vi "Create Serial Output Channel CSI-2 IO x8.vi"() -> (4 "serial output channel io x8":T4)   [LabVIEW 2020, in "GettingStarted_Gen_148X_FPGA.lvlib"]
uses:
  GettingStarted_Gen_148X_FPGA.lvlib
  Common/Types/Serial Output Channel IO.ctl
  Common/Types/Serial Output Channel IO 32b.ctl
  Common/Types/Serial Output Channel IO 64b.ctl
  Common/GettingStarted_Common_148X_FPGA.lvlib
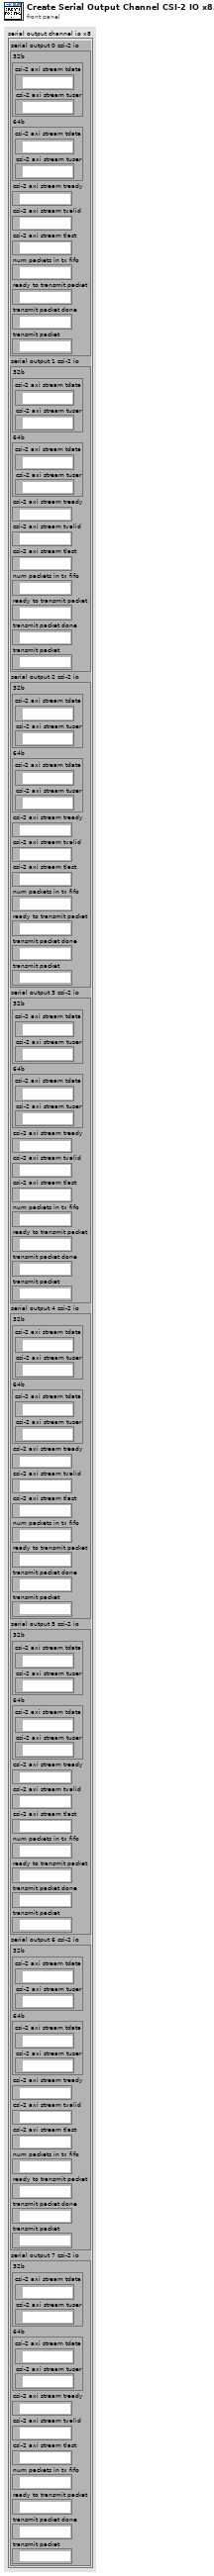
[diagram p1: front panel]
types:
  T1 = typedef "GettingStarted_Common_148X_FPGA.lvlib/Serial Output Channel IO.ctl" = cluster{"32b":T2, "64b":T3, "csi-2 axi stream tready":refnum<k21>, "csi-2 axi stream tvalid":refnum<k21>, "csi-2 axi stream tlast":refnum<k21>, "num packets in tx fifo":refnum<k21>, "ready to transmit packet":refnum<k21>, "transmit packet done":refnum<k21>, "transmit packet":refnum<k21>}
  T2 = typedef "GettingStarted_Common_148X_FPGA.lvlib/Serial Output Channel IO 32b.ctl" = cluster{"csi-2 axi stream tdata":refnum<k21>, "csi-2 axi stream tuser":refnum<k21>}
  T3 = typedef "GettingStarted_Common_148X_FPGA.lvlib/Serial Output Channel IO 64b.ctl" = cluster{"csi-2 axi stream tdata":refnum<k21>, "csi-2 axi stream tuser":refnum<k21>}
  T4 = cluster{"serial output 0 csi-2 io":T1, "serial output 1 csi-2 io":T1, "serial output 2 csi-2 io":T1, "serial output 3 csi-2 io":T1, "serial output 4 csi-2 io":T1, "serial output 5 csi-2 io":T1, "serial output 6 csi-2 io":T1, "serial output 7 csi-2 io":T1}
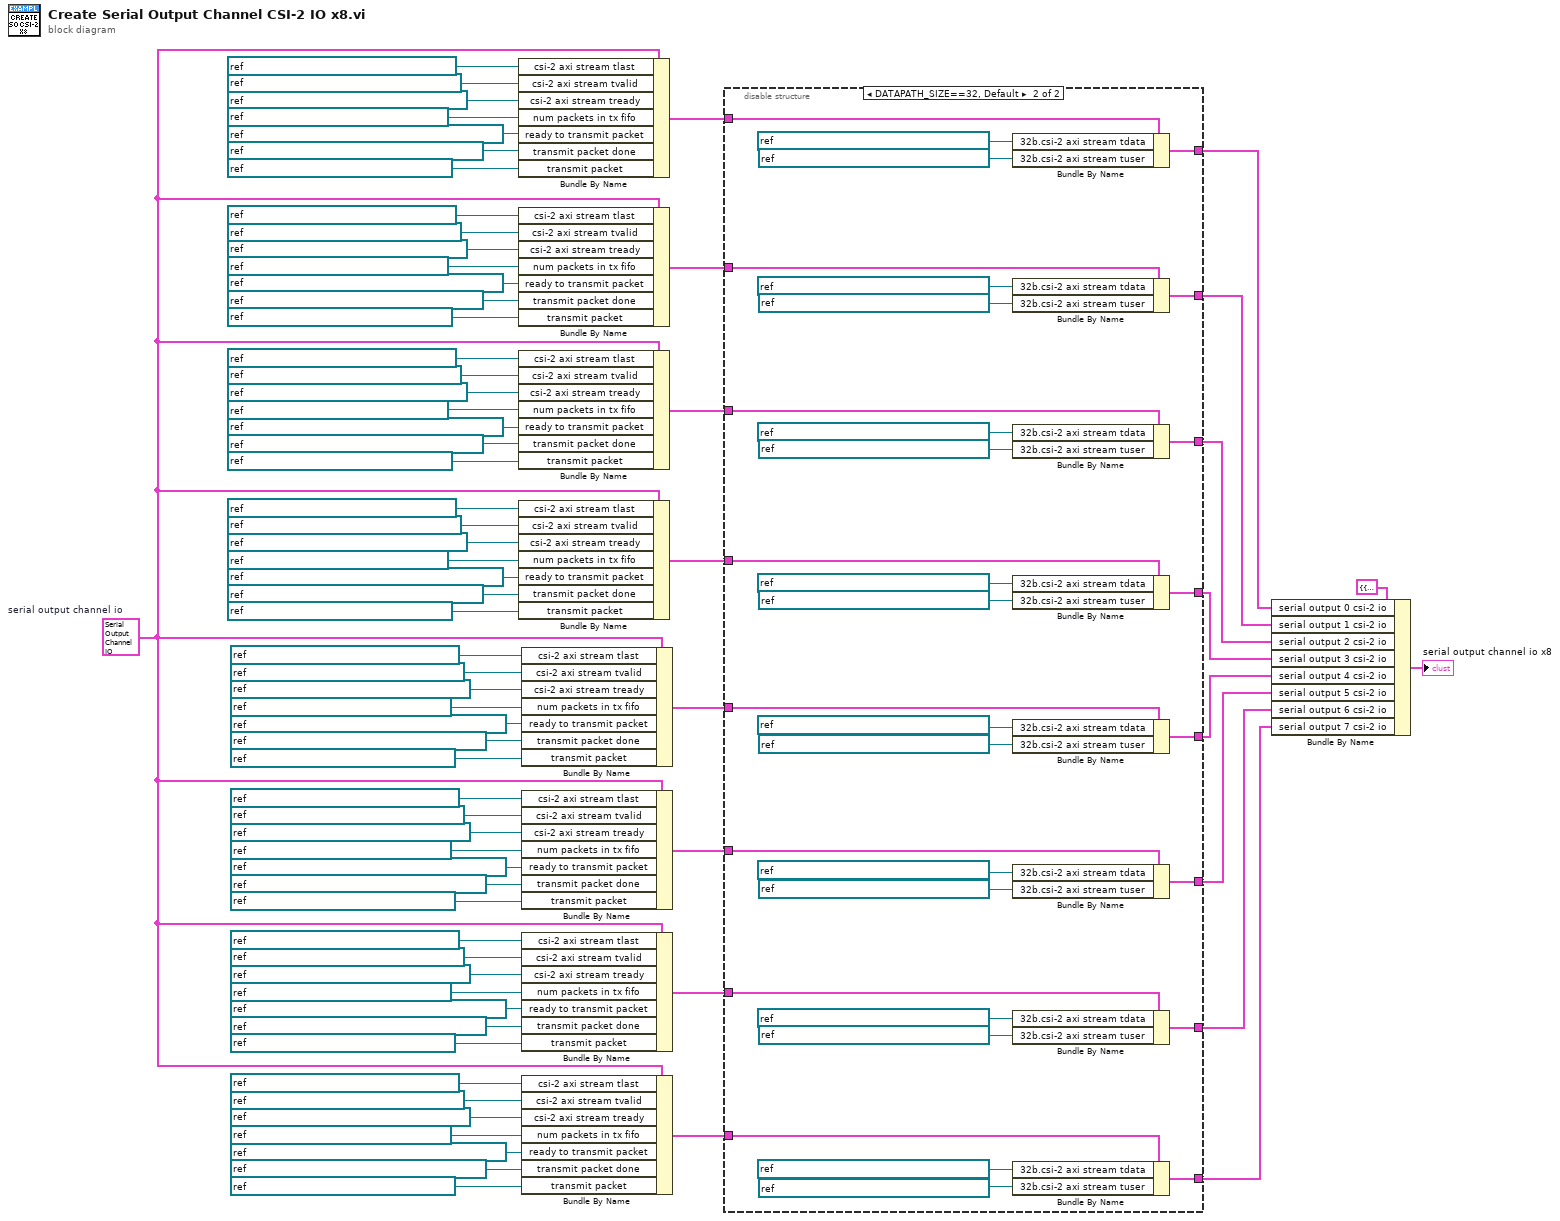
[diagram p0: block diagram]
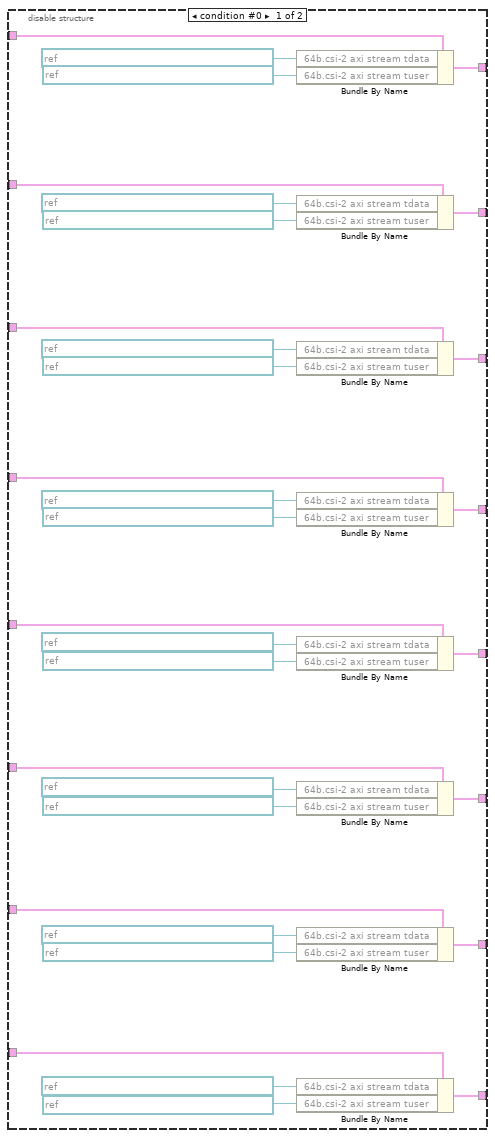
[diagram p2: hidden frame]
diagram:
  w21 = T1 {"32b"={"csi-2 axi stream tdata"="", "csi-2 axi stream tuser"=""}, "64b"={"csi-2 axi stream tdata"="", "csi-2 axi stream tuser"=""}, "csi-2 axi stream tready"="", "csi-2 axi stream tvalid"="", "csi-2 axi stream tlast"="", "num packets in tx fifo"="", "ready to transmit packet"="", "transmit packet done"="", "transmit packet"=""}  # serial output channel io
  n1 = Bundle By Name(cluster=w21, "csi-2 axi stream tlast"=refnum<k21> "IO Socket\\SO 0 CSI-2 AXI Stream TLast", "csi-2 axi stream tvalid"=refnum<k21> "IO Socket\\SO 0 CSI-2 AXI Stream TValid", "csi-2 axi stream tready"=refnum<k21> "IO Socket\\SO 0 CSI-2 AXI Stream TReady", "num packets in tx fifo"=refnum<k21> "IO Socket\\SO 0 CSI-2 Packets In FIFO", "ready to transmit packet"=refnum<k21> "IO Socket\\SO 0 CSI-2 Ready To Transmit Packet", "transmit packet done"=refnum<k21> "IO Socket\\SO 0 CSI-2 Transmit Packet Done", "transmit packet"=refnum<k21> "IO Socket\\SO 0 CSI-2 Transmit Packet") -> (w25:T1)
  n2 = Bundle By Name(cluster=w21, "csi-2 axi stream tlast"=refnum<k21> "IO Socket\\SO 1 CSI-2 AXI Stream TLast", "csi-2 axi stream tvalid"=refnum<k21> "IO Socket\\SO 1 CSI-2 AXI Stream TValid", "csi-2 axi stream tready"=refnum<k21> "IO Socket\\SO 1 CSI-2 AXI Stream TReady", "num packets in tx fifo"=refnum<k21> "IO Socket\\SO 1 CSI-2 Packets In FIFO", "ready to transmit packet"=refnum<k21> "IO Socket\\SO 1 CSI-2 Ready To Transmit Packet", "transmit packet done"=refnum<k21> "IO Socket\\SO 1 CSI-2 Transmit Packet Done", "transmit packet"=refnum<k21> "IO Socket\\SO 1 CSI-2 Transmit Packet") -> (w24:T1)
  n3 = Bundle By Name(cluster=w21, "csi-2 axi stream tlast"=refnum<k21> "IO Socket\\SO 2 CSI-2 AXI Stream TLast", "csi-2 axi stream tvalid"=refnum<k21> "IO Socket\\SO 2 CSI-2 AXI Stream TValid", "csi-2 axi stream tready"=refnum<k21> "IO Socket\\SO 2 CSI-2 AXI Stream TReady", "num packets in tx fifo"=refnum<k21> "IO Socket\\SO 2 CSI-2 Packets In FIFO", "ready to transmit packet"=refnum<k21> "IO Socket\\SO 2 CSI-2 Ready To Transmit Packet", "transmit packet done"=refnum<k21> "IO Socket\\SO 2 CSI-2 Transmit Packet Done", "transmit packet"=refnum<k21> "IO Socket\\SO 2 CSI-2 Transmit Packet") -> (w23:T1)
  n4 = Bundle By Name(cluster=w21, "csi-2 axi stream tlast"=refnum<k21> "IO Socket\\SO 3 CSI-2 AXI Stream TLast", "csi-2 axi stream tvalid"=refnum<k21> "IO Socket\\SO 3 CSI-2 AXI Stream TValid", "csi-2 axi stream tready"=refnum<k21> "IO Socket\\SO 3 CSI-2 AXI Stream TReady", "num packets in tx fifo"=refnum<k21> "IO Socket\\SO 3 CSI-2 Packets In FIFO", "ready to transmit packet"=refnum<k21> "IO Socket\\SO 3 CSI-2 Ready To Transmit Packet", "transmit packet done"=refnum<k21> "IO Socket\\SO 3 CSI-2 Transmit Packet Done", "transmit packet"=refnum<k21> "IO Socket\\SO 3 CSI-2 Transmit Packet") -> (w22:T1)
  n5 = Bundle By Name(cluster=w21, "csi-2 axi stream tlast"=refnum<k21> "IO Socket\\SO 4 CSI-2 AXI Stream TLast", "csi-2 axi stream tvalid"=refnum<k21> "IO Socket\\SO 4 CSI-2 AXI Stream TValid", "csi-2 axi stream tready"=refnum<k21> "IO Socket\\SO 4 CSI-2 AXI Stream TReady", "num packets in tx fifo"=refnum<k21> "IO Socket\\SO 4 CSI-2 Packets In FIFO", "ready to transmit packet"=refnum<k21> "IO Socket\\SO 4 CSI-2 Ready To Transmit Packet", "transmit packet done"=refnum<k21> "IO Socket\\SO 4 CSI-2 Transmit Packet Done", "transmit packet"=refnum<k21> "IO Socket\\SO 4 CSI-2 Transmit Packet") -> (w12:T1)
  n6 = Bundle By Name(cluster=w21, "csi-2 axi stream tlast"=refnum<k21> "IO Socket\\SO 5 CSI-2 AXI Stream TLast", "csi-2 axi stream tvalid"=refnum<k21> "IO Socket\\SO 5 CSI-2 AXI Stream TValid", "csi-2 axi stream tready"=refnum<k21> "IO Socket\\SO 5 CSI-2 AXI Stream TReady", "num packets in tx fifo"=refnum<k21> "IO Socket\\SO 5 CSI-2 Packets In FIFO", "ready to transmit packet"=refnum<k21> "IO Socket\\SO 5 CSI-2 Ready To Transmit Packet", "transmit packet done"=refnum<k21> "IO Socket\\SO 5 CSI-2 Transmit Packet Done", "transmit packet"=refnum<k21> "IO Socket\\SO 5 CSI-2 Transmit Packet") -> (w11:T1)
  n7 = Bundle By Name(cluster=w21, "csi-2 axi stream tlast"=refnum<k21> "IO Socket\\SO 6 CSI-2 AXI Stream TLast", "csi-2 axi stream tvalid"=refnum<k21> "IO Socket\\SO 6 CSI-2 AXI Stream TValid", "csi-2 axi stream tready"=refnum<k21> "IO Socket\\SO 6 CSI-2 AXI Stream TReady", "num packets in tx fifo"=refnum<k21> "IO Socket\\SO 6 CSI-2 Packets In FIFO", "ready to transmit packet"=refnum<k21> "IO Socket\\SO 6 CSI-2 Ready To Transmit Packet", "transmit packet done"=refnum<k21> "IO Socket\\SO 6 CSI-2 Transmit Packet Done", "transmit packet"=refnum<k21> "IO Socket\\SO 6 CSI-2 Transmit Packet") -> (w10:T1)
  n8 = Bundle By Name(cluster=w21, "csi-2 axi stream tlast"=refnum<k21> "IO Socket\\SO 7 CSI-2 AXI Stream TLast", "csi-2 axi stream tvalid"=refnum<k21> "IO Socket\\SO 7 CSI-2 AXI Stream TValid", "csi-2 axi stream tready"=refnum<k21> "IO Socket\\SO 7 CSI-2 AXI Stream TReady", "num packets in tx fifo"=refnum<k21> "IO Socket\\SO 7 CSI-2 Packets In FIFO", "ready to transmit packet"=refnum<k21> "IO Socket\\SO 7 CSI-2 Ready To Transmit Packet", "transmit packet done"=refnum<k21> "IO Socket\\SO 7 CSI-2 Transmit Packet Done", "transmit packet"=refnum<k21> "IO Socket\\SO 7 CSI-2 Transmit Packet") -> (w9:T1)
  n9 = disable-structure shown="DATAPATH_SIZE==32, Default" {
    disable-tunnel: [w93 w133] -> w6
    disable-tunnel: [w92 w132] -> w3
    disable-tunnel: [w95 w135] -> w4
    disable-tunnel: [w94 w134] -> w5
    disable-tunnel: w25 -> [w103 w139]
    disable-tunnel: w24 -> [w102 w138]
    disable-tunnel: w23 -> [w101 w137]
    disable-tunnel: w22 -> [w100 w136]
    disable-tunnel: w12 -> [w83 w123]
    disable-tunnel: w11 -> [w81 w122]
    disable-tunnel: w10 -> [w80 w121]
    disable-tunnel: w9 -> [w79 w120]
    disable-tunnel: [w82 w119] -> w7
    disable-tunnel: [w78 w118] -> w8
    disable-tunnel: [w77 w117] -> w2
    disable-tunnel: [w76 w116] -> w1
    frame condition #0 {
      n10 = Bundle By Name(cluster=w103, "64b.csi-2 axi stream tdata"=refnum<k21> "IO Socket\\SO 0 CSI-2 AXI Stream TData" ("csi-2 axi stream tdata"), "64b.csi-2 axi stream tuser"=refnum<k21> "IO Socket\\SO 0 CSI-2 AXI Stream TUser" ("csi-2 axi stream tuser")) -> (w92:T1)
      n11 = Bundle By Name(cluster=w102, "64b.csi-2 axi stream tdata"=refnum<k21> "IO Socket\\SO 1 CSI-2 AXI Stream TData" ("csi-2 axi stream tdata"), "64b.csi-2 axi stream tuser"=refnum<k21> "IO Socket\\SO 1 CSI-2 AXI Stream TUser" ("csi-2 axi stream tuser")) -> (w95:T1)
      n12 = Bundle By Name(cluster=w101, "64b.csi-2 axi stream tdata"=refnum<k21> "IO Socket\\SO 2 CSI-2 AXI Stream TData" ("csi-2 axi stream tdata"), "64b.csi-2 axi stream tuser"=refnum<k21> "IO Socket\\SO 2 CSI-2 AXI Stream TUser" ("csi-2 axi stream tuser")) -> (w94:T1)
      n13 = Bundle By Name(cluster=w100, "64b.csi-2 axi stream tdata"=refnum<k21> "IO Socket\\SO 3 CSI-2 AXI Stream TData" ("csi-2 axi stream tdata"), "64b.csi-2 axi stream tuser"=refnum<k21> "IO Socket\\SO 3 CSI-2 AXI Stream TUser" ("csi-2 axi stream tuser")) -> (w93:T1)
      n14 = Bundle By Name(cluster=w83, "64b.csi-2 axi stream tdata"=refnum<k21> "IO Socket\\SO 4 CSI-2 AXI Stream TData" ("csi-2 axi stream tdata"), "64b.csi-2 axi stream tuser"=refnum<k21> "IO Socket\\SO 4 CSI-2 AXI Stream TUser" ("csi-2 axi stream tuser")) -> (w82:T1)
      n15 = Bundle By Name(cluster=w81, "64b.csi-2 axi stream tdata"=refnum<k21> "IO Socket\\SO 5 CSI-2 AXI Stream TData" ("csi-2 axi stream tdata"), "64b.csi-2 axi stream tuser"=refnum<k21> "IO Socket\\SO 5 CSI-2 AXI Stream TUser" ("csi-2 axi stream tuser")) -> (w78:T1)
      n16 = Bundle By Name(cluster=w80, "64b.csi-2 axi stream tdata"=refnum<k21> "IO Socket\\SO 6 CSI-2 AXI Stream TData" ("csi-2 axi stream tdata"), "64b.csi-2 axi stream tuser"=refnum<k21> "IO Socket\\SO 6 CSI-2 AXI Stream TUser" ("csi-2 axi stream tuser")) -> (w77:T1)
      n17 = Bundle By Name(cluster=w79, "64b.csi-2 axi stream tdata"=refnum<k21> "IO Socket\\SO 7 CSI-2 AXI Stream TData" ("csi-2 axi stream tdata"), "64b.csi-2 axi stream tuser"=refnum<k21> "IO Socket\\SO 7 CSI-2 AXI Stream TUser" ("csi-2 axi stream tuser")) -> (w76:T1)
    }
    frame condition #1 (active) {
      n18 = Bundle By Name(cluster=w139, "32b.csi-2 axi stream tdata"=refnum<k21> "IO Socket\\SO 0 CSI-2 AXI Stream TData" ("csi-2 axi stream tdata"), "32b.csi-2 axi stream tuser"=refnum<k21> "IO Socket\\SO 0 CSI-2 AXI Stream TUser" ("csi-2 axi stream tuser")) -> (w132:T1)
      n19 = Bundle By Name(cluster=w138, "32b.csi-2 axi stream tdata"=refnum<k21> "IO Socket\\SO 1 CSI-2 AXI Stream TData" ("csi-2 axi stream tdata"), "32b.csi-2 axi stream tuser"=refnum<k21> "IO Socket\\SO 1 CSI-2 AXI Stream TUser" ("csi-2 axi stream tuser")) -> (w135:T1)
      n20 = Bundle By Name(cluster=w137, "32b.csi-2 axi stream tdata"=refnum<k21> "IO Socket\\SO 2 CSI-2 AXI Stream TData" ("csi-2 axi stream tdata"), "32b.csi-2 axi stream tuser"=refnum<k21> "IO Socket\\SO 2 CSI-2 AXI Stream TUser" ("csi-2 axi stream tuser")) -> (w134:T1)
      n21 = Bundle By Name(cluster=w136, "32b.csi-2 axi stream tdata"=refnum<k21> "IO Socket\\SO 3 CSI-2 AXI Stream TData" ("csi-2 axi stream tdata"), "32b.csi-2 axi stream tuser"=refnum<k21> "IO Socket\\SO 3 CSI-2 AXI Stream TUser" ("csi-2 axi stream tuser")) -> (w133:T1)
      n22 = Bundle By Name(cluster=w123, "32b.csi-2 axi stream tdata"=refnum<k21> "IO Socket\\SO 4 CSI-2 AXI Stream TData" ("csi-2 axi stream tdata"), "32b.csi-2 axi stream tuser"=refnum<k21> "IO Socket\\SO 4 CSI-2 AXI Stream TUser" ("csi-2 axi stream tuser")) -> (w119:T1)
      n23 = Bundle By Name(cluster=w122, "32b.csi-2 axi stream tdata"=refnum<k21> "IO Socket\\SO 5 CSI-2 AXI Stream TData" ("csi-2 axi stream tdata"), "32b.csi-2 axi stream tuser"=refnum<k21> "IO Socket\\SO 5 CSI-2 AXI Stream TUser" ("csi-2 axi stream tuser")) -> (w118:T1)
      n24 = Bundle By Name(cluster=w121, "32b.csi-2 axi stream tdata"=refnum<k21> "IO Socket\\SO 6 CSI-2 AXI Stream TData" ("csi-2 axi stream tdata"), "32b.csi-2 axi stream tuser"=refnum<k21> "IO Socket\\SO 6 CSI-2 AXI Stream TUser" ("csi-2 axi stream tuser")) -> (w117:T1)
      n25 = Bundle By Name(cluster=w120, "32b.csi-2 axi stream tdata"=refnum<k21> "IO Socket\\SO 7 CSI-2 AXI Stream TData" ("csi-2 axi stream tdata"), "32b.csi-2 axi stream tuser"=refnum<k21> "IO Socket\\SO 7 CSI-2 AXI Stream TUser" ("csi-2 axi stream tuser")) -> (w116:T1)
    }
  }
  n26 = Bundle By Name(cluster=T4 {"serial output 0 csi-2 io"={"32b"={"csi-2 axi stream tdata"="", "csi-2 axi stream tuser"=""}, "64b"={"csi-2 axi stream tdata"="", "csi-2 axi stream tuser"=""}, "csi-2 axi stream tready"="", "csi-2 axi stream tvalid"="", "csi-2 axi stream tlast"="", "num packets in tx fifo"="", "ready to transmit packet"="", "transmit packet done"="", "transmit packet"=""}, "serial output 1 csi-2 io"={"32b"={"csi-2 axi stream tdata"="", "csi-2 axi stream tuser"=""}, "64b"={"csi-2 axi stream tdata"="", "csi-2 axi stream tuser"=""}, "csi-2 axi stream tready"="", "csi-2 axi stream tvalid"="", "csi-2 axi stream tlast"="", "num packets in tx fifo"="", "ready to transmit packet"="", "transmit packet done"="", "transmit packet"=""}, "serial output 2 csi-2 io"={"32b"={"csi-2 axi stream tdata"="", "csi-2 axi stream tuser"=""}, "64b"={"csi-2 axi stream tdata"="", "csi-2 axi stream tuser"=""}, "csi-2 axi stream tready"="", "csi-2 axi stream tvalid"="", "csi-2 axi stream tlast"="", "num packets in tx fifo"="", "ready to transmit packet"="", "transmit packet done"="", "transmit packet"=""}, "serial output 3 csi-2 io"={"32b"={"csi-2 axi stream tdata"="", "csi-2 axi stream tuser"=""}, "64b"={"csi-2 axi stream tdata"="", "csi-2 axi stream tuser"=""}, "csi-2 axi stream tready"="", "csi-2 axi stream tvalid"="", "csi-2 axi stream tlast"="", "num packets in tx fifo"="", "ready to transmit packet"="", "transmit packet done"="", "transmit packet"=""}, "serial output 4 csi-2 io"={"32b"={"csi-2 axi stream tdata"="", "csi-2 axi stream tuser"=""}, "64b"={"csi-2 axi stream tdata"="", "csi-2 axi stream tuser"=""}, "csi-2 axi stream tready"="", "csi-2 axi stream tvalid"="", "csi-2 axi stream tlast"="", "num packets in tx fifo"="", "ready to transmit packet"="", "transmit packet done"="", "transmit packet"=""}, "serial output 5 csi-2 io"={"32b"={"csi-2 axi stream tdata"="", "csi-2 axi stream tuser"=""}, "64b"={"csi-2 axi stream tdata"="", "csi-2 axi stream tuser"=""}, "csi-2 axi stream tready"="", "csi-2 axi stream tvalid"="", "csi-2 axi stream tlast"="", "num packets in tx fifo"="", "ready to transmit packet"="", "transmit packet done"="", "transmit packet"=""}, "serial output 6 csi-2 io"={"32b"={"csi-2 axi stream tdata"="", "csi-2 axi stream tuser"=""}, "64b"={"csi-2 axi stream tdata"="", "csi-2 axi stream tuser"=""}, "csi-2 axi stream tready"="", "csi-2 axi stream tvalid"="", "csi-2 axi stream tlast"="", "num packets in tx fifo"="", "ready to transmit packet"="", "transmit packet done"="", "transmit packet"=""}, "serial output 7 csi-2 io"={"32b"={"csi-2 axi stream tdata"="", "csi-2 axi stream tuser"=""}, "64b"={"csi-2 axi stream tdata"="", "csi-2 axi stream tuser"=""}, "csi-2 axi stream tready"="", "csi-2 axi stream tvalid"="", "csi-2 axi stream tlast"="", "num packets in tx fifo"="", "ready to transmit packet"="", "transmit packet done"="", "transmit packet"=""}} ("serial output channel io x4"), "serial output 0 csi-2 io"=w3, "serial output 1 csi-2 io"=w4, "serial output 2 csi-2 io"=w5, "serial output 3 csi-2 io"=w6, "serial output 4 csi-2 io"=w7, "serial output 5 csi-2 io"=w8, "serial output 6 csi-2 io"=w2, "serial output 7 csi-2 io"=w1) -> (→"serial output channel io x8":T4)
